vi "test program.vi"() -> ()   [LabVIEW 2016]
uses:
  <vilib>/SmarAct/MCS/Types/mcsPacket.ctl
  test state machine.ctl
panel:
  in  "Home":bool
  in  "revolution":i32
  in  "ROTATE":bool
  in  "MOVE XY":bool
  out "arrived angle":bool
  in  "angle difference abs":i32
  out "state":enum16{"idle", "running", "fault"}(ring)
  out "arrived xy":bool
  out "packet":T1
  in  "Position Difference y [nm]":i32=8000
  in  "Position Difference x [nm]":i32=8000
  out "Error":errorcluster
  in  "pause":bool
  out "Exit":bool
  out "connected":bool
  in  "connect":bool
  in  "findSystems":bool caption="Find Systems"
  in  "System locator":string(combo)
  in  "start":bool
  # "A linear positioner with integrated sensor \nshould be connected to channel 0."
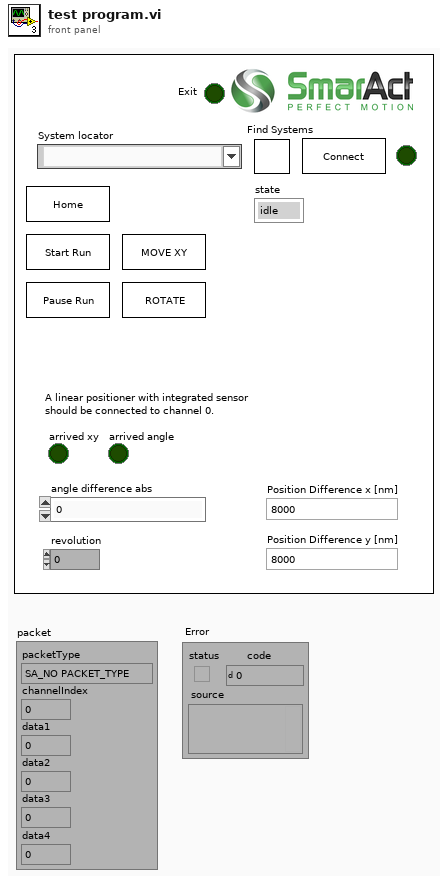
[diagram p1: front panel]
types:
  T1 = typedef "mcsPacket.ctl" = cluster{"packetType":enum32{"SA_NO PACKET_TYPE", "SA_ERROR_ PACKET_TYPE", "SA_POSITION PACKET_TYPE", "SA_COMPLETED PACKET_TYPE", "SA_STATUS PACKET_TYPE", "SA_ANGLE_PACKET_TYPE", "SA_VOLTAGE_LEVEL_PACKET_TYPE", "SA_SENSOR_TYPE_PACKET_TYPE", "SA_SENSOR_ENABLED_PACKET_TYPE", "SA_END_EFFECTOR_TYPE_PACKET_TYPE", "SA_GRIPPER_OPENING_PACKET_TYPE", "SA_FORCE_PACKET_TYPE", "SA_MOVE_SPEED_PACKET_TYPE", "SA_PHYSICAL_POSITION_KNOWN_PACKET_TYPE", "SA_POSITION_LIMIT_PACKET_TYPE", "SA_ANGLE_LIMIT_PACKET_TYPE", "SA_SAFE_DIRECTION_PACKET_TYPE", "SA_SCALE_PACKET_TYPE", "SA_MOVE_ACCELERATION_PACKET_TYPE", "SA_CHANNEL_PROPERTY_PACKET_TYPE", "SA_CAPTURE_BUFFER_PACKET_TYPE", "SA_TRIGGERED_PACKET_TYPE"}, "channelIndex":u32, "data1":u32, "data2":i32, "data3":i32, "data4":u32}
  T2 = typedef "test state machine.ctl" = enum16{"ARRIVED_ROTATE", "ROTATE", "GOTO_XY", "IDLE", "START", "STOP", "ARRIVED_XY", ""}
  T3 = enum32{"SA_NO PACKET_TYPE", "SA_ERROR_ PACKET_TYPE", "SA_POSITION PACKET_TYPE", "SA_COMPLETED PACKET_TYPE", "SA_STATUS PACKET_TYPE", "SA_ANGLE_PACKET_TYPE", "SA_VOLTAGE_LEVEL_PACKET_TYPE", "SA_SENSOR_TYPE_PACKET_TYPE", "SA_SENSOR_ENABLED_PACKET_TYPE", "SA_END_EFFECTOR_TYPE_PACKET_TYPE", "SA_GRIPPER_OPENING_PACKET_TYPE", "SA_FORCE_PACKET_TYPE", "SA_MOVE_SPEED_PACKET_TYPE", "SA_PHYSICAL_POSITION_KNOWN_PACKET_TYPE", "SA_POSITION_LIMIT_PACKET_TYPE", "SA_ANGLE_LIMIT_PACKET_TYPE", "SA_SAFE_DIRECTION_PACKET_TYPE", "SA_SCALE_PACKET_TYPE", "SA_MOVE_ACCELERATION_PACKET_TYPE", "SA_CHANNEL_PROPERTY_PACKET_TYPE", "SA_CAPTURE_BUFFER_PACKET_TYPE", "SA_TRIGGERED_PACKET_TYPE"}
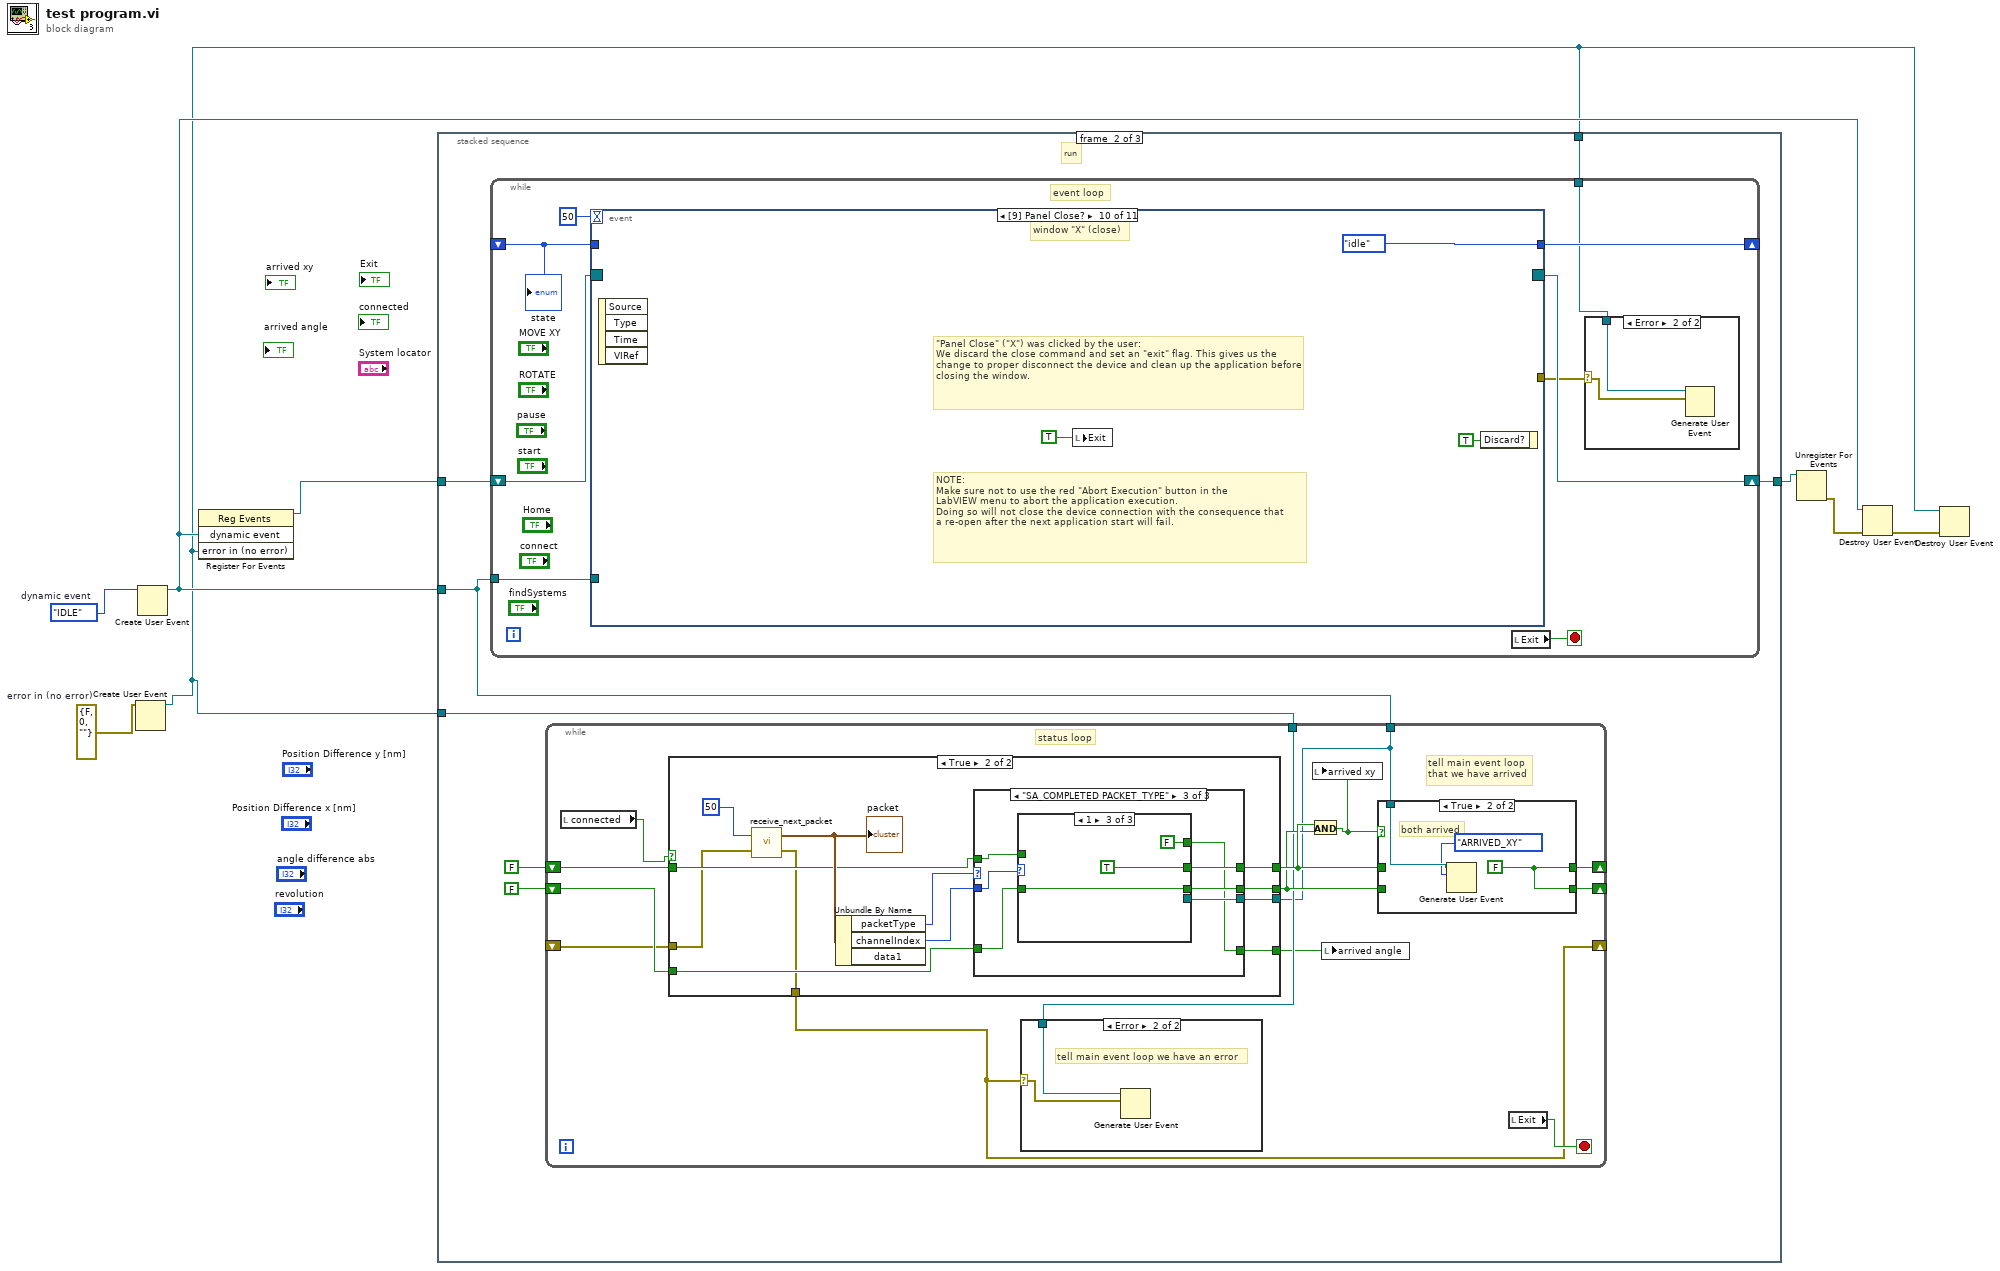
[diagram p0: block diagram]
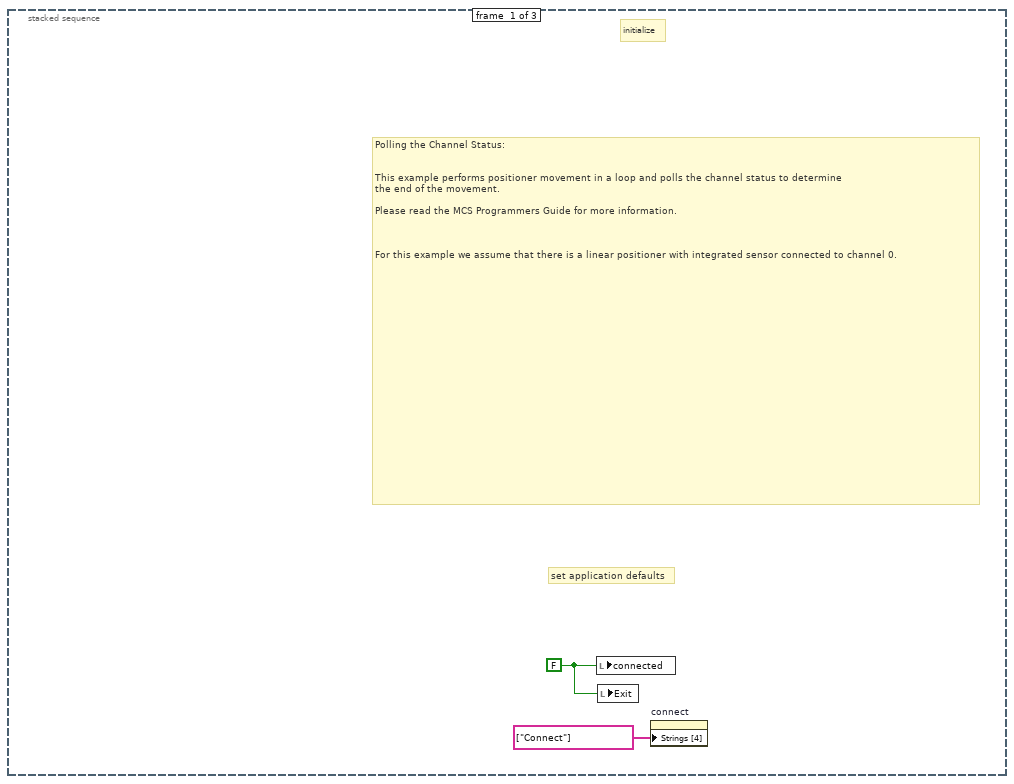
[diagram p2: hidden frame]
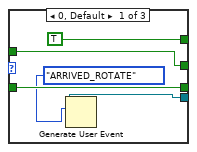
[diagram p8: hidden frame]
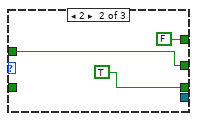
[diagram p9: hidden frame]
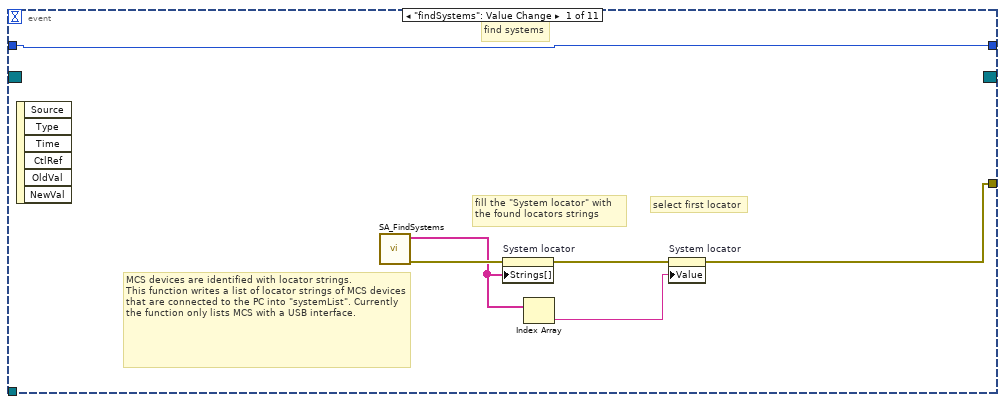
[diagram p11: hidden frame]
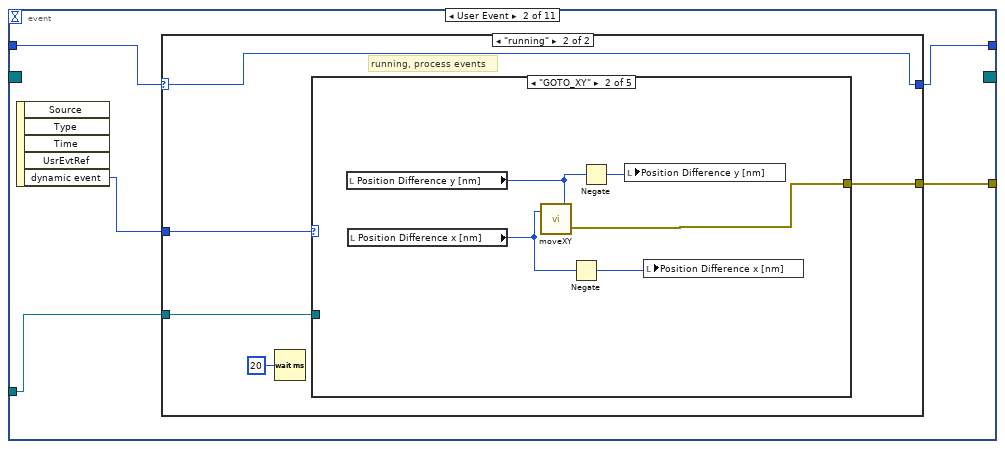
[diagram p12: hidden frame]
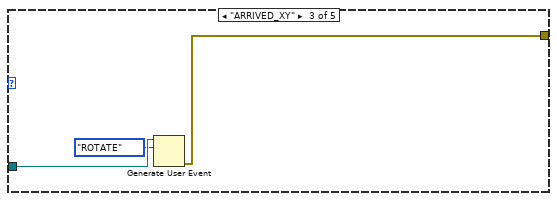
[diagram p15: hidden frame]
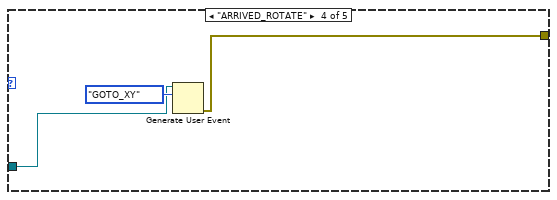
[diagram p16: hidden frame]
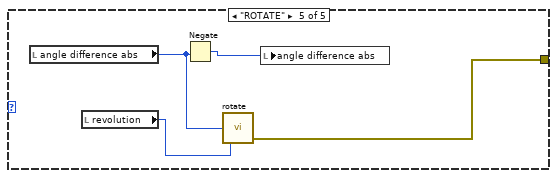
[diagram p17: hidden frame]
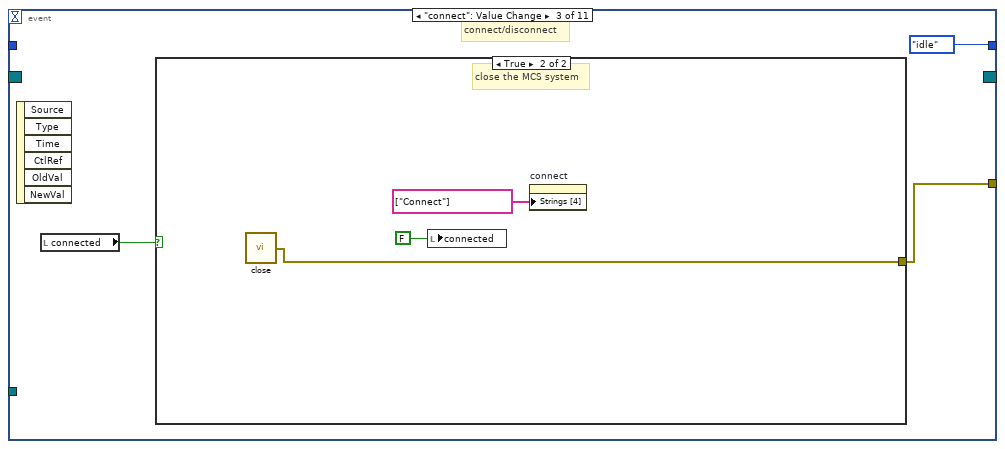
[diagram p18: hidden frame]
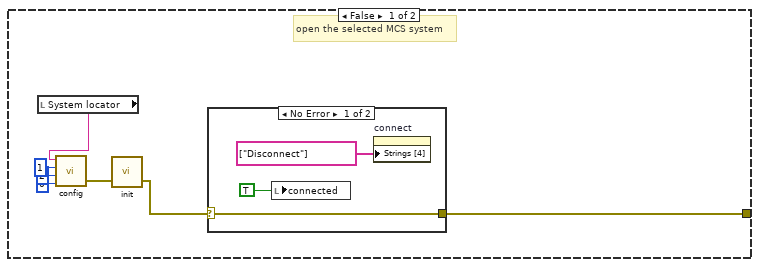
[diagram p19: hidden frame]
diagram:
  w3 = errorcluster {"status"=FALSE, "code"=0, "source"=""}  # error in (no error)
  w5 = test_state_machine."IDLE"  # dynamic event
  n1 = Create User Event(user event datatype=w3) -> (user event=w1:refnum<user-event>)  [unwired: 1 in, 1 out]
  n2 = Create User Event(user event datatype=w5) -> (user event=w4:refnum<user-event>)  [unwired: 1 in, 1 out]
  n3 = register-events(w4, w1) -> (reference out=w8:refnum<event-registration>)  [unwired: 2 in, 1 out]
  n4 = stacked-sequence {
    tunnel: w8 -> [_ w15 _]
    tunnel: [_ w14 _] -> w7
    tunnel: w4 -> [_ w13 _]
    tunnel: w1 -> [_ w12 _]
    tunnel: w1 -> [_ w11 _]
    frame #0 {
      w10 = FALSE ("connected")
      # "Polling the Channel Status:\n\n\nThis example performs positioner movement in a loop and polls the channel status to determine\nthe end of the movement.\n\nPlease read the MCS Programmers Guide for more information.\n\n\n\nFor this example we assume that there is a linear positioner with integrated sensor connected to channel 0."
      # "set application defaults"
      # "initialize"
      n5 = local write "connected"(w10) -> ()
      n6 = local write "Exit"(w10) -> ()
      n7 = property on="connect" class="Bool"("Strings [4]"=string[] ["Connect"]) -> ()  [unwired: 2 in, 2 out]
    }
    frame #1 {
      # "run"
      n8 = while {
        shift-right: [w80] -> w14
        shift-left: w15 -> [w81]
        tunnel: w13 -> [w79]
        shift-right: [w77] -> _
        shift-left: _ -> [w78]
        tunnel: w11 -> [w75]
        stop <- w82 stop-if-true
        # "event loop"
        n9 = event shown="[9] Panel Close?" {
          selector: w81 -> [_ _ _ _ _ _ _ _ _ _ _]
          dyn-events: [_ _ _ _ _ _ _ _ _ _ _] -> w80
          timeout: 50 -> [_ _ _ _ _ _ _ _ _ _ _]
          tunnel: w79 -> [_ w95 _ _ w138 _ _ _ _ _ _]
          tunnel: w78 -> [w87 w94 _ _ _ _ _ _ _ _ w160]
          tunnel: [w87 w93 enum16{"idle", "running", "fault"}."idle" ("state") enum16{"idle", "running", "fault"}."idle" ("state") enum16{"idle", "running", "fault"}."running" ("state") _ _ enum16{"idle", "running", "fault"}."idle" ("state") _ enum16{"idle", "running", "fault"}."idle" ("state") w160] -> w77
          tunnel: [w86 w92 w118 _ _ _ _ _ _ _ _] -> w76
          event "findSystems": Value Change {
            # "select first locator"
            # "fill the \"System locator\" with\nthe found locators strings"
            # "MCS devices are identified with locator strings.\nThis function writes a list of locator strings of MCS devices that are connected to the PC into \"systemList\". Currently the function only lists MCS with a USB interface."
            # "find systems"
            n10 = event-data() -> ()  [unwired: 1 in, 6 out]
            n11 = call <vilib>:"SA_FindSystems.vi"() -> ("error out"=w91:errorcluster, "systemList"=w90:string[])  [unwired: 10 in]
            n12 = property on="System locator" class="CmbBox"(error in=w91, "Strings[]"=w90) -> (error out=w89:errorcluster)  [unwired: 1 in, 1 out]
            n13 = Index Array(array=w90) -> (element=w88:string)  [unwired: 1 in]
            n14 = property on="System locator" class="CmbBox"(error in=w89, "Value"=w88) -> (error out=w86:errorcluster)  [unwired: 1 in, 1 out]
          }
          event User Event {
            n15 = event-data() -> ("dynamic event"=w96:T2)  [unwired: 1 in, 4 out]
            n16 = case shown="\"running\"" w94 {
              selector: w94 -> [w97 w100]
              tunnel: w96 -> [_ w102]
              tunnel: w95 -> [_ w101]
              tunnel: [w97 w100] -> w93
              tunnel: [_ w98] -> w92
              frame "idle", Default {
                # "idle, remain idle, don't respond to events"
              }
              frame "running" {
                # "running, process events"
                n17 = Wait (ms)(milliseconds to wait=u32 20) -> ()  [unwired: 1 out]
                n18 = case shown="\"GOTO_XY\"" w102 {
                  tunnel: w101 -> [_ _ w110 w112 _]
                  tunnel: [_ w103 w108 w111 w114] -> w98
                  frame "IDLE", Default {
                  }
                  frame "GOTO_XY" {
                    n19 = local read "Position Difference y [nm]"() -> (w104:i32)
                    n20 = local read "Position Difference x [nm]"() -> (w106:i32)
                    n21 = call "moveXY.vi"("y position"=w104, "x position"=w106) -> ("error out"=w103:errorcluster)  [unwired: 1 in]
                    n22 = Negate(x=w106) -> (-x=w107:i32)
                    n23 = Negate(x=w104) -> (-x=w105:i32)
                    n24 = local write "Position Difference y [nm]"(w105) -> ()
                    n25 = local write "Position Difference x [nm]"(w107) -> ()
                  }
                  frame "ARRIVED_XY" {
                    n26 = Generate User Event(user event=w110, event data cluster=test_state_machine."ROTATE" ("event data")) -> (error out=w108:errorcluster)  [unwired: 2 in, 1 out]
                  }
                  frame "ARRIVED_ROTATE" {
                    n27 = Generate User Event(user event=w112, event data cluster=test_state_machine."GOTO_XY" ("event data")) -> (error out=w111:errorcluster)  [unwired: 2 in, 1 out]
                  }
                  frame "ROTATE" {
                    n28 = local read "angle difference abs"() -> (w115:i32)
                    n29 = local read "revolution"() -> (w117:i32)
                    n30 = Negate(x=w115) -> (-x=w116:i32)
                    n31 = call "rotate.vi"("angle"=w115, "revolution"=w117) -> ("error out"=w114:errorcluster)  [unwired: 3 in]
                    n32 = local write "angle difference abs"(w116) -> ()
                  }
                }
              }
            }
          }
          event "connect": Value Change {
            # "connect/disconnect"
            n33 = event-data() -> ()  [unwired: 1 in, 6 out]
            n34 = local read "connected"() -> (w120:bool)
            n35 = case shown="True" w120 {
              tunnel: [w127 w132] -> w118
              frame False {
                # "open the selected MCS system"
                n36 = local read "System locator"() -> (w125:string)
                n37 = call "config.vi"("System locator"=w125, "X channel"=u32 1, "Y channel"=u32 2, "Rotation channel"=u32 0) -> ("error out"=w126:errorcluster)  [unwired: 1 in]
                n38 = call "init.vi"("error in (no error)"=w126) -> ("error out"=w121:errorcluster)  [unwired: 2 in]
                n39 = case shown="No Error" w121 {
                  selector: w121 -> [w128 w131]
                  tunnel: [w128 w131] -> w127
                  frame No Error {
                    n40 = local write "connected"(TRUE ("connected")) -> ()
                    n41 = property on="connect" class="Bool"("Strings [4]"=string[] ["Disconnect"]) -> ()  [unwired: 2 in, 2 out]
                  }
                  frame Error {
                  }
                }
              }
              frame True {
                # "close the MCS system"
                n42 = call "close.vi"() -> ("error out"=w132:errorcluster)  [unwired: 1 in]
                n43 = local write "connected"(FALSE ("connected")) -> ()
                n44 = property on="connect" class="Bool"("Strings [4]"=string[] ["Connect"]) -> ()  [unwired: 2 in, 2 out]
              }
            }
          }
          event "pause": Value Change {
            # "stop"
            n45 = event-data() -> ()  [unwired: 1 in, 6 out]
            n46 = local read "connected"() -> (w136:bool)
            n47 = case shown="True" w136 {
              frame False {
              }
              frame True {
                n48 = call "stop.vi"() -> ()  [unwired: 1 in, 1 out]
              }
            }
          }
          event "start": Value Change {
            # "start move loop"
            n49 = event-data() -> ()  [unwired: 1 in, 6 out]
            n50 = local read "connected"() -> (w139:bool)
            n51 = case shown="True" w139 {
              tunnel: w138 -> [_ w141]
              frame False {
              }
              frame True {
                n52 = Generate User Event(user event=w141, event data cluster=test_state_machine."GOTO_XY" ("event data")) -> ()  [unwired: 2 in, 2 out]
              }
            }
          }
          event "MOVE XY": Value Change {
            # "manually move xy"
            n53 = event-data() -> ()  [unwired: 1 in, 6 out]
            n54 = local read "Position Difference y [nm]"() -> (w143:i32)
            n55 = local read "Position Difference x [nm]"() -> (w145:i32)
            n56 = call "moveXY.vi"("y position"=w143, "x position"=w145) -> ("error out"=w142:errorcluster)  [unwired: 1 in]
            n57 = Negate(x=w145) -> (-x=w146:i32)
            n58 = Negate(x=w143) -> (-x=w144:i32)
            n59 = local write "Position Difference y [nm]"(w144) -> ()
            n60 = local write "Position Difference x [nm]"(w146) -> ()
            n61 = local write "Error"(w142) -> ()
          }
          event "ROTATE": Value Change {
            # "manually rotate"
            n62 = event-data() -> ()  [unwired: 1 in, 6 out]
            n63 = local read "angle difference abs"() -> (w147:i32)
            n64 = local read "revolution"() -> (w149:i32)
            n65 = Negate(x=w147) -> (-x=w148:i32)
            n66 = call "rotate.vi"("angle"=w147, "revolution"=w149) -> ()  [unwired: 3 in, 1 out]
            n67 = local write "angle difference abs"(w148) -> ()
          }
          event User Event {
            # "error in polling loop"
            n68 = event-data() -> ("status"=w150:bool, "code"=w151:i32, "source"=w152:string)  [unwired: 1 in, 4 out]
            n69 = Bundle By Name(cluster=errorcluster {"status"=FALSE, "code"=0, "source"=""} ("Error"), "status"=w150, "code"=w151, "source"=w152) -> (w154:errorcluster)
            n70 = call <vilib>:"Simple Error Handler.vi"("error in (no error)"=w154) -> ("error out"=→"Error":errorcluster)  [unwired: 4 in, 4 out]
          }
          event "Home": Value Change {
            # "home xy and rotation to a known starting point"
            n71 = event-data() -> ()  [unwired: 1 in, 6 out]
          }
          event Panel Close? {
            # "NOTE:\nMake sure not to use the red \"Abort Execution\" button in the\nLabVIEW menu to abort the application execution.\nDoing so will not close the device connection with the consequence that\na re-open after the next application start will fail."
            # "\"Panel Close\" (\"X\") was clicked by the user:\nWe discard the close command and set an \"exit\" flag. This gives us the change to proper disconnect the device and clean up the application before closing the window."
            # "window \"X\" (close)"
            n72 = event-data() -> ()  [unwired: 1 in, 4 out]
            n73 = local write "Exit"(TRUE ("exit")) -> ()
            n74 = event-data("Discard?"=TRUE) -> ()  [unwired: 1 in, 1 out]
          }
          event Timeout {
            # "update display"
            n75 = event-data() -> ()  [unwired: 1 in, 3 out]
          }
        }
        n76 = local read "Exit"() -> (w82:bool)
        n77 = case shown="Error" w76 {
          selector: w76 -> [_ w85]
          tunnel: w75 -> [_ w84]
          frame No Error {
          }
          frame Error {
            n78 = Generate User Event(user event=w84, event data cluster=w85) -> ()  [unwired: 2 in, 2 out]
          }
        }
        "state" <- w78
      }
      n79 = while {
        shift-right: [w28] -> _
        shift-left: FALSE -> [w30]
        shift-right: [w26] -> _
        shift-left: FALSE -> [w29]
        tunnel: w13 -> [w20]
        tunnel: w12 -> [w24]
        shift-right: [w22] -> _
        shift-left: _ -> [w23]
        stop <- w31 stop-if-true
        # "tell main event loop\nthat we have arrived"
        # "status loop"
        n80 = local read "connected"() -> (w21:bool)
        n81 = case shown="True" w21 {
          tunnel: [w40 w48] -> w27
          tunnel: w30 -> [w40 w47]
          tunnel: [w39 w46] -> w25
          tunnel: w29 -> [w39 w45]
          tunnel: [_ w44] -> w22
          tunnel: w23 -> [_ w43]
          tunnel: w20 -> [_ w42]
          tunnel: [_ w41] -> w18
          frame False {
            # "no error"
          }
          frame True {
            n82 = call "receive_next_packet.vi"("error in (no error)"=w43, "timeout"=u32 50) -> ("error out"=w44:errorcluster, "packet"=w51:T1)
            "packet" <- w51
            n83 = Unbundle By Name(w51) -> ("packetType"=w50:T3, "channelIndex"=w49:u32)  [unwired: 1 out]
            n84 = case shown="\"SA_COMPLETED PACKET_TYPE\"" w50 {
              tunnel: w49 -> [_ _ w62]
              tunnel: [w54 w56 w63] -> w48
              tunnel: w47 -> [w54 w56 w61]
              tunnel: [w53 w55 w60] -> w46
              tunnel: w45 -> [w53 w55 w59]
              tunnel: w42 -> [_ _ w58]
              tunnel: [_ _ w57] -> w41
              frame "SA_NO PACKET_TYPE", Default {
              }
              frame "SA_ERROR_ PACKET_TYPE" {
              }
              frame "SA_COMPLETED PACKET_TYPE" {
                n85 = case shown="1" w62 {
                  tunnel: [w67 w70 TRUE] -> w63
                  tunnel: w61 -> [w67 w70 _]
                  tunnel: [w68 TRUE w73] -> w60
                  tunnel: w59 -> [w68 _ w73]
                  tunnel: w58 -> [w66 _ _]
                  tunnel: [TRUE ("arrived angle") FALSE ("arrived angle") FALSE ("arrived angle")] -> w57
                  frame 0, Default {
                    n86 = Generate User Event(user event=w66, event data cluster=test_state_machine."ARRIVED_ROTATE" ("event data")) -> ()  [unwired: 2 in, 2 out]
                  }
                  frame 2 {
                  }
                  frame 1 {
                  }
                }
              }
            }
          }
        }
        n87 = case shown="Error" w22 {
          selector: w22 -> [_ w33]
          tunnel: w24 -> [_ w32]
          frame No Error {
          }
          frame Error {
            # "tell main event loop we have an error"
            n88 = Generate User Event(user event=w32, event data cluster=w33) -> ()  [unwired: 2 in, 2 out]
          }
        }
        n89 = And(x=w27, y=w25) -> (x .and. y?=w19:bool)
        n90 = local write "arrived xy"(w19) -> ()
        n91 = local write "arrived angle"(w18) -> ()
        n92 = case shown="True" w19 {
          tunnel: [w35 w38] -> w28
          tunnel: w27 -> [w35 _]
          tunnel: [w34 w38] -> w26
          tunnel: w25 -> [w34 _]
          tunnel: w20 -> [_ w37]
          frame False {
          }
          frame True {
            w38 = FALSE
            # "both arrived"
            n93 = Generate User Event(user event=w37, event data cluster=test_state_machine."ARRIVED_XY" ("event data")) -> ()  [unwired: 2 in, 2 out]
          }
        }
        n94 = local read "Exit"() -> (w31:bool)
      }
    }
    frame #2 {
      # "clean up"
      n95 = local read "connected"() -> (w161:bool)
      n96 = case shown="True" w161 {
        frame False {
        }
        frame True {
          # "always make sure to close the connection\nto the device before quitting the program"
          n97 = call "close.vi"() -> ("error out"=w162:errorcluster)  [unwired: 1 in]
          n98 = call <vilib>:"Clear Errors.vi"("error in (no error)"=w162) -> ()  [unwired: 5 in, 2 out]
        }
      }
    }
  }
  n99 = Unregister For Events(event registration refnum=w7) -> (error out=w6:errorcluster)  [unwired: 1 in]
  n100 = Destroy User Event(user event=w4, error in=w6) -> (error out=w2:errorcluster)
  n101 = Destroy User Event(user event=w1, error in=w2) -> ()  [unwired: 1 out]
